vi "ELVIS III v1.0 Shutdown Writing DMA.vi"(8 "error in (no error)":errorcluster) -> (0 "error out":errorcluster)   [LabVIEW 2021]
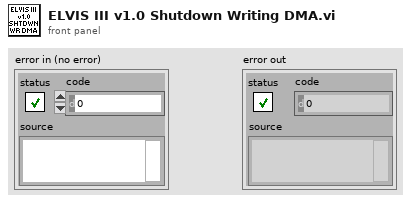
[diagram p1: front panel]
types:
  T1 = typedef "Block Write Resource.ctl" = refnum<vi>
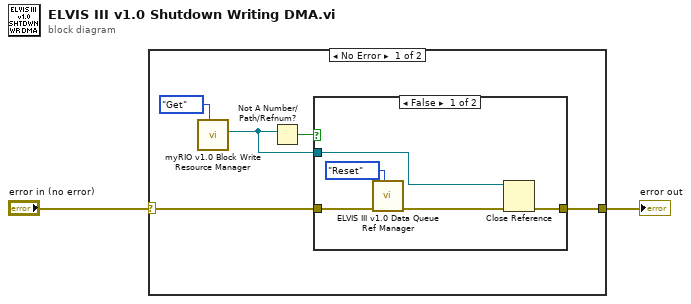
[diagram p0: block diagram]
diagram:
  n1 = case shown="No Error" "error in (no error)" {
    selector: "error in (no error)" -> [w5 w14]
    tunnel: [w4 w14] -> w1
    frame No Error {
      n2 = call <vilib>:"myRIO v1.0 Block Write Resource Manager.vi"("Action"=enum16{"Get", "Set", "Reset"}."Get") -> ("Resource Data Out"=w3:T1)  [unwired: 10 in]
      n3 = Not A Number/Path/Refnum?(number/path/refnum=w3) -> (NaN/Path/Refnum?=w6:bool)
      n4 = case shown="False" w6 {
        tunnel: w3 -> [w9 _]
        tunnel: w5 -> [w12 w13]
        tunnel: [w11 w13] -> w4
        frame False {
          n5 = call <vilib>:"ELVIS III v1.0 Data Queue Ref Manager.vi"("Action"=enum16{"Get", "Reset"}."Reset", "error in (no error)"=w12) -> ("error out"=w8:errorcluster)  [unwired: 7 in, 1 out]
          n6 = Close Reference(reference=w9, error in (no error)=w8) -> (error out=w11:errorcluster)
        }
        frame True {
        }
      }
    }
    frame Error {
    }
  }
  "error out" <- w1
